vi "PhysMon-Default Options.vi"(11 "error in (no error)":errorcluster) -> (8 "Options":T1={"Min Interval"=0.0, "HR from ABR?"=FALSE, "HR Scale"={"Slope"=0.0, "Offset"=0.0, "Limits"={"Min"=0.0, "Max"=0.0}, "term config"=-1}, "Temp Scale"={"Slope"=0.0, "Offset"=0.0, "Limits"={"Min"=0.0, "Max"=0.0}, "term config"=-1}, "Lock?"=TRUE, "Temp Sensor"=enum."YSI", "EKG"={"Sample duration (s)"=0.0}} {"Temp Scale"."term config" items=["default"=-1, "RSE"=10083, "NRSE"=10078, "Differential"=10106, "Pseudodifferential"=12529]; "HR Scale"."term config" items=["default"=-1, "RSE"=10083, "NRSE"=10078, "Differential"=10106, "Pseudodifferential"=12529]}, 15 "error out":errorcluster)   [LabVIEW 2020]
uses:
  Typedefs/PhysMon-Options.ctl
  Typedefs/PhysMon-Scale.ctl
  Typedefs/PhysMon-TempSensor.ctl
  Typedefs/PhysMon-HR From EKG Settings.ctl
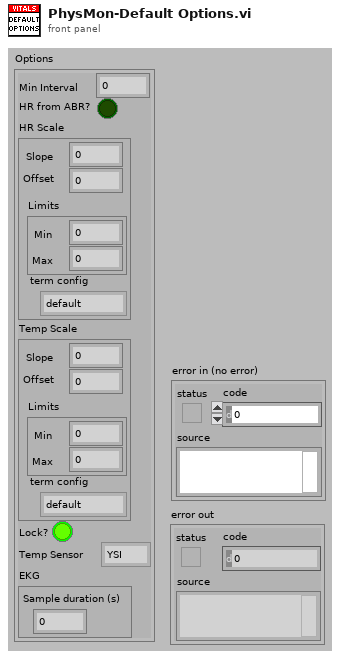
[diagram p1: front panel]
types:
  T1 = typedef "PhysMon-Options.ctl" = cluster{"Min Interval":dbl, "HR from ABR?":bool, "HR Scale":T2, "Temp Scale":T2, "Lock?":bool, "Temp Sensor":T3, "EKG":T4}
  T2 = typedef "PhysMon-Scale.ctl" = cluster{"Slope":dbl, "Offset":dbl, "Limits":cluster{"Min":dbl, "Max":dbl}, "term config":i32}
  T3 = typedef "PhysMon-TempSensor.ctl" = enum16{"YSI", "FHC", "Custom"}
  T4 = typedef "PhysMon-HR From EKG Settings.ctl" = cluster{"Sample duration (s)":dbl}
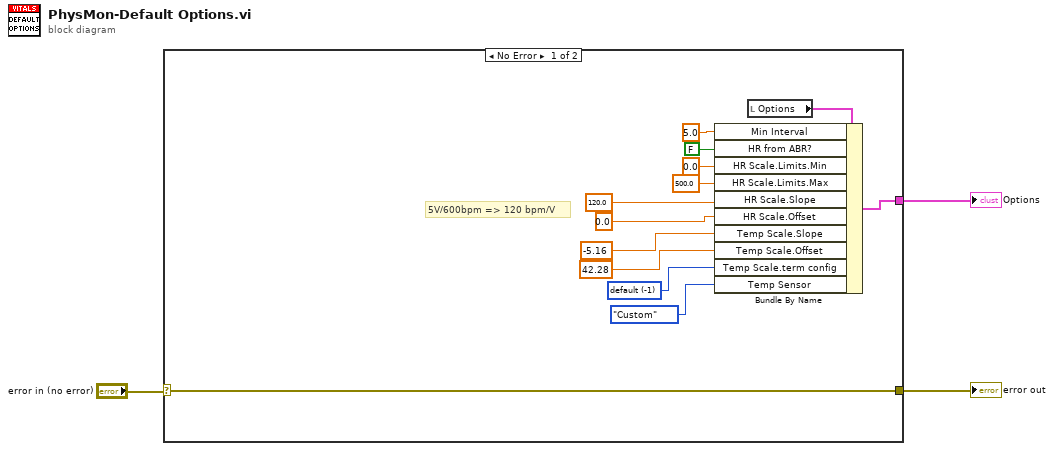
[diagram p0: block diagram]
diagram:
  n1 = case shown="No Error" "error in (no error)" {
    selector: "error in (no error)" -> [w16 w17]
    tunnel: [w16 w17] -> w2
    tunnel: [w14 _] -> w1
    frame No Error {
      w5 = -1 items=["default"=-1, "RSE"=10083, "NRSE"=10078, "Differential"=10106, "Pseudodifferential"=12529] ("input terminal configuration")
      # "5V/600bpm => 120 bpm/V"
      n2 = local read "Options"() -> (w15:T1)
      n3 = Bundle By Name(cluster=w15, "Min Interval"=5.0, "HR from ABR?"=FALSE, "HR Scale.Limits.Min"=0.0, "HR Scale.Limits.Max"=500.0, "HR Scale.Slope"=120.0 ("y"), "HR Scale.Offset"=0.0 ("y"), "Temp Scale.Slope"=-5.16 ("y"), "Temp Scale.Offset"=42.28 ("y"), "Temp Scale.term config"=w5, "Temp Sensor"=PhysMon-TempSensor."Custom") -> (w14:T1)
    }
    frame Error {
    }
  }
  "error out" <- w2
  "Options" <- w1
